vi "Request - Should Read Body.vi"() -> (3 "Unit Test Framework Results":T1)   [LabVIEW 2023, in "Request.lvclass"]
doc: "Use this template to create a user-defined test VI. Define your test requirements and wire the results to the <b>Result (Test)</b> control. Do not modify the <b>Unit Test Framework Results</b> indicator."
uses:
  Request.lvclass
  <vilib>/utf/common/utf_test_comparison_operators.ctl
  <vilib>/utf/NI_UnitTestFramework.lvlib
  <vilib>/utf/common/utf_test_result.ctl
  <vilib>/utf/common/utf_test_result_failure.ctl
  <vilib>/utf/common/utf_test_result_troll.ctl
  <vilib>/utf/common/utf_vi_tag.ctl
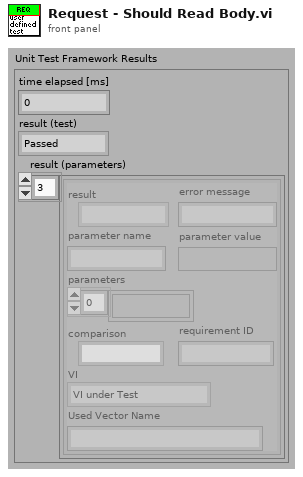
[diagram p1: front panel]
types:
  T1 = typedef "NI_UnitTestFramework.lvlib/utf_test_result_troll.ctl" = cluster{"time elapsed [ms]":u32, "result (test)":T2, "result (parameters)":T3[]}
  T2 = typedef "NI_UnitTestFramework.lvlib/utf_test_result.ctl" = enum16{"Passed", "Failed", "Error", "Skipped", "Not Processed"}
  T3 = typedef "NI_UnitTestFramework.lvlib/utf_test_result_failure.ctl" = cluster{"result":T2, "error message":string, "parameter name":string, "parameter value":variant, "parameters":variant[], "comparison":T4, "requirement ID":string, "VI":T5, "Used Vector Name":string}
  T4 = typedef "NI_UnitTestFramework.lvlib/utf_test_comparison_operators.ctl" = enum16{"=", "!=", ">", ">=", "<", "<=", "range", "symmetric tolerance", "asymmetric tolerance", "string contains", "string not contain", "array size", "string length", "array range", "by element", "array range (limit array)", "user-defined", "array contains", "array not contain", "vector length", "= (elm)", "!= (elm)", "= (case insensitive)", "!= (case insensitive)"}
  T5 = typedef "NI_UnitTestFramework.lvlib/utf_vi_tag.ctl" = enum16{"Setup VI", "VI under Test", "Teardown VI"}
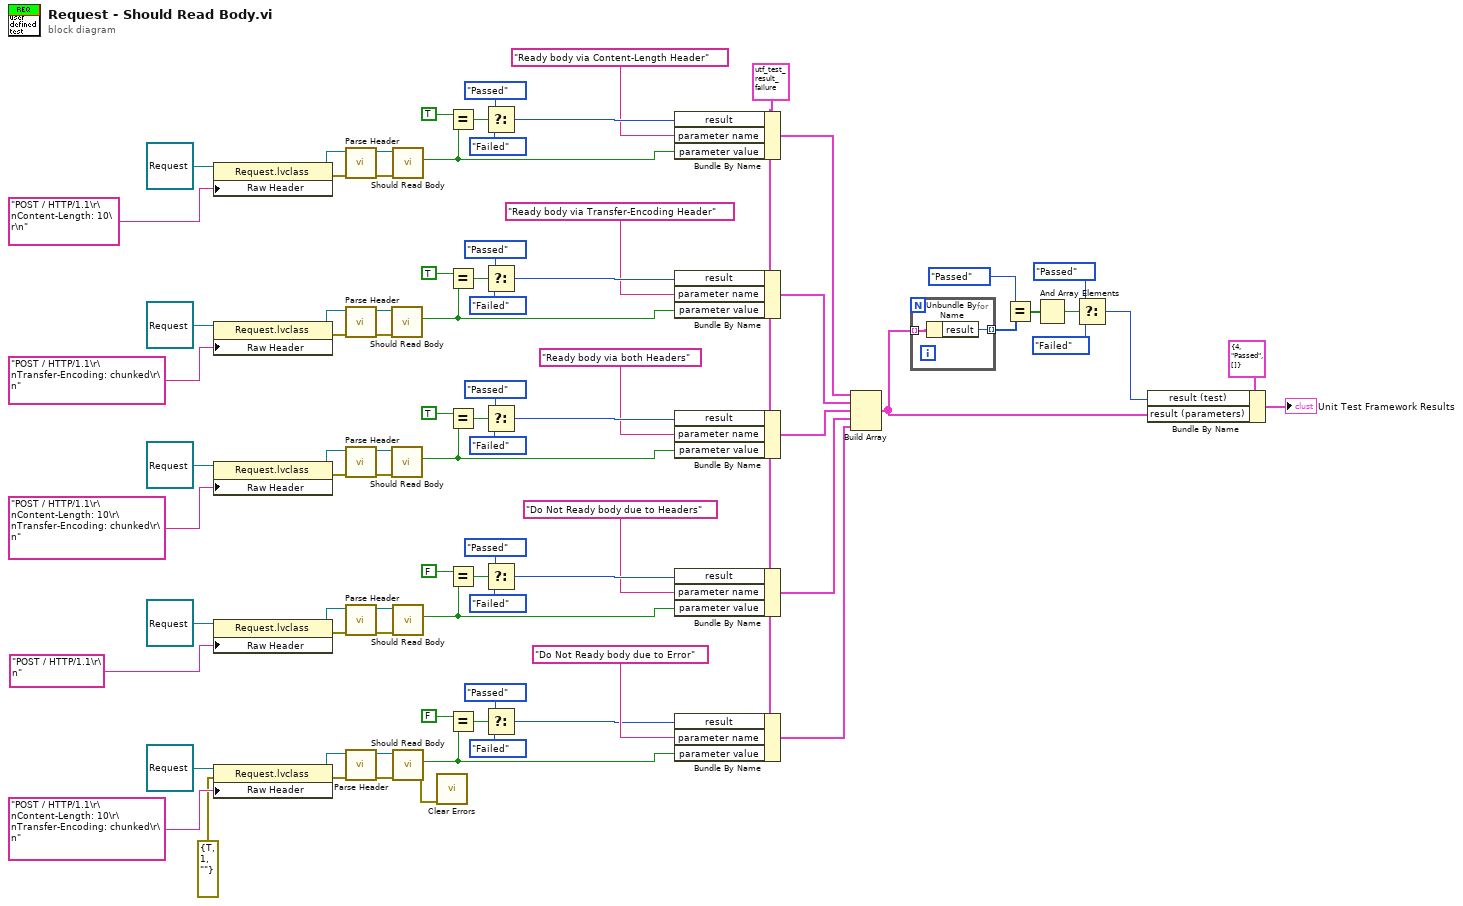
[diagram p0: block diagram]
diagram:
  w5 = T3 {"result"=enum."Not Processed", "error message"="", "parameter name"="", "parameter value"=variant, "parameters"=[], "comparison"=enum."=", "requirement ID"="", "VI"=enum."VI under Test", "Used Vector Name"=""} ("Unit Test Framework - result (parameters)")
  n1 = property class="Request.lvclass"(reference=refnum<class "Request.lvclass"> refnum ("Request.lvclass"), "Raw Header"="POST / HTTP/1.1\r\nContent-Length: 10\r\n") -> (reference out=w80:refnum<class "Request.lvclass">, error out=w79:errorcluster)  [unwired: 1 in]
  n2 = property class="Request.lvclass"(reference=refnum<class "Request.lvclass"> refnum ("Request.lvclass"), "Raw Header"="POST / HTTP/1.1\r\nTransfer-Encoding: chunked\r\n") -> (reference out=w50:refnum<class "Request.lvclass">, error out=w51:errorcluster)  [unwired: 1 in]
  n3 = property class="Request.lvclass"(reference=refnum<class "Request.lvclass"> refnum ("Request.lvclass"), "Raw Header"="POST / HTTP/1.1\r\nContent-Length: 10\r\nTransfer-Encoding: chunked\r\n") -> (reference out=w47:refnum<class "Request.lvclass">, error out=w46:errorcluster)  [unwired: 1 in]
  n4 = property class="Request.lvclass"(reference=refnum<class "Request.lvclass"> refnum ("Request.lvclass"), "Raw Header"="POST / HTTP/1.1\r\n") -> (reference out=w24:refnum<class "Request.lvclass">, error out=w25:errorcluster)  [unwired: 1 in]
  n5 = property class="Request.lvclass"(reference=refnum<class "Request.lvclass"> refnum ("Request.lvclass"), error in=errorcluster {"status"=TRUE, "code"=1, "source"=""} ("error in (no error)"), "Raw Header"="POST / HTTP/1.1\r\nContent-Length: 10\r\nTransfer-Encoding: chunked\r\n") -> (reference out=w15:refnum<class "Request.lvclass">, error out=w14:errorcluster)
  n6 = call "Parse Header.vi"("error in (no error)"=w79, "Request in"=w80) -> ("error out"=w65:errorcluster, "Request out"=w64:refnum<class "Request.lvclass">)  [unwired: 8 in]
  n7 = call "Parse Header.vi"("error in (no error)"=w51, "Request in"=w50) -> ("error out"=w56:errorcluster, "Request out"=w57:refnum<class "Request.lvclass">)  [unwired: 8 in]
  n8 = call "Parse Header.vi"("error in (no error)"=w46, "Request in"=w47) -> ("error out"=w41:errorcluster, "Request out"=w40:refnum<class "Request.lvclass">)  [unwired: 8 in]
  n9 = call "Parse Header.vi"("error in (no error)"=w25, "Request in"=w24) -> ("error out"=w30:errorcluster, "Request out"=w31:refnum<class "Request.lvclass">)  [unwired: 8 in]
  n10 = call "Parse Header.vi"("error in (no error)"=w14, "Request in"=w15) -> ("error out"=w2:errorcluster, "Request out"=w9:refnum<class "Request.lvclass">)  [unwired: 8 in]
  n11 = call "Should Read Body.vi"("error in (no error)"=w56, "Request in"=w57) -> ("Read Body?"=w59:bool)  [unwired: 7 in, 2 out]
  n12 = call "Should Read Body.vi"("error in (no error)"=w41, "Request in"=w40) -> ("Read Body?"=w38:bool)  [unwired: 7 in, 2 out]
  n13 = call "Should Read Body.vi"("error in (no error)"=w65, "Request in"=w64) -> ("Read Body?"=w62:bool)  [unwired: 7 in, 2 out]
  n14 = call "Should Read Body.vi"("error in (no error)"=w30, "Request in"=w31) -> ("Read Body?"=w33:bool)  [unwired: 7 in, 2 out]
  n15 = call "Should Read Body.vi"("error in (no error)"=w2, "Request in"=w9) -> ("error out"=w3:errorcluster, "Read Body?"=w7:bool)  [unwired: 7 in, 1 out]
  n16 = call <vilib>:"Clear Errors.vi"("error in (no error)"=w3) -> ()  [unwired: 5 in, 2 out]
  n17 = Equal?(x=TRUE, y=w62) -> (x = y?=w77:bool)
  n18 = Equal?(x=TRUE, y=w59) -> (x = y?=w52:bool)
  n19 = Equal?(x=TRUE, y=w38) -> (x = y?=w45:bool)
  n20 = Equal?(x=FALSE, y=w33) -> (x = y?=w26:bool)
  n21 = Equal?(x=FALSE, y=w7) -> (x = y?=w13:bool)
  n22 = Select(t=utf_test_result."Passed" ("result"), s=w77, f=utf_test_result."Failed" ("result")) -> (s? t:f=w76:T2)
  n23 = Select(t=utf_test_result."Passed" ("result"), s=w52, f=utf_test_result."Failed" ("result")) -> (s? t:f=w53:T2)
  n24 = Select(t=utf_test_result."Passed" ("result"), s=w45, f=utf_test_result."Failed" ("result")) -> (s? t:f=w44:T2)
  n25 = Select(t=utf_test_result."Passed" ("result"), s=w26, f=utf_test_result."Failed" ("result")) -> (s? t:f=w27:T2)
  n26 = Select(t=utf_test_result."Passed" ("result"), s=w13, f=utf_test_result."Failed" ("result")) -> (s? t:f=w12:T2)
  n27 = Bundle By Name(cluster=w5, "result"=w76, "parameter name"="Ready body via Content-Length Header", "parameter value"=w62) -> (w78:T3)
  n28 = Bundle By Name(cluster=w5, "result"=w53, "parameter name"="Ready body via Transfer-Encoding Header", "parameter value"=w59) -> (w36:T3)
  n29 = Bundle By Name(cluster=w5, "result"=w44, "parameter name"="Ready body via both Headers", "parameter value"=w38) -> (w35:T3)
  n30 = Bundle By Name(cluster=w5, "result"=w27, "parameter name"="Do Not Ready body due to Headers", "parameter value"=w33) -> (w22:T3)
  n31 = Bundle By Name(cluster=w5, "result"=w12, "parameter name"="Do Not Ready body due to Error", "parameter value"=w7) -> (w4:T3)
  n32 = Build Array(w78, w36, w35, w22, w4) -> (w73:T3[])
  n33 = for {
    tunnel: w73 -> [w85] mode=indexing
    tunnel: [w84] -> w72 mode=indexing
    n34 = Unbundle By Name(w85) -> ("result"=w84:T2)
  }
  n35 = Equal?(x=utf_test_result."Passed" ("result"), y=w72) -> (x = y?=w70:bool[])
  n36 = And Array Elements(Boolean array=w70) -> (logical AND=w69:bool)
  n37 = Select(t=utf_test_result."Passed" ("result"), s=w69, f=utf_test_result."Failed" ("result")) -> (s? t:f=w66:T2)
  n38 = Bundle By Name(cluster=T1 {"time elapsed [ms]"=4, "result (test)"=enum."Passed", "result (parameters)"=[]} ("Unit Test Framework - Result"), "result (test)"=w66, "result (parameters)"=w73) -> (→"Unit Test Framework Results":T1)
